vi "Create Sequence File.vi"(8 "error in (no error)":errorcluster, 11 "niRFSTS Sequence Flow in":refnum<class "niRFSTS Sequence Flow.lvclass">) -> (0 "error out":errorcluster, 3 "niRFSTS Sequence Flow out":refnum<class "niRFSTS Sequence Flow.lvclass">)   [LabVIEW 2018, in "niRFSTS Sequence Flow.lvclass"]
uses:
  niRFSTS Sequence Flow.lvclass
  niRFSTS Sequence Flow.lvclass/niRFSTS Sequence Flow.ctl
  Plugins/TestStand API Tools (TSAT).lvlibp/Sequence File Actions/TSAT Sequence File Actions.lvlib
  Plugins/TestStand API Tools (TSAT).lvlibp/TSAT Examples/TSAT Examples.lvlib
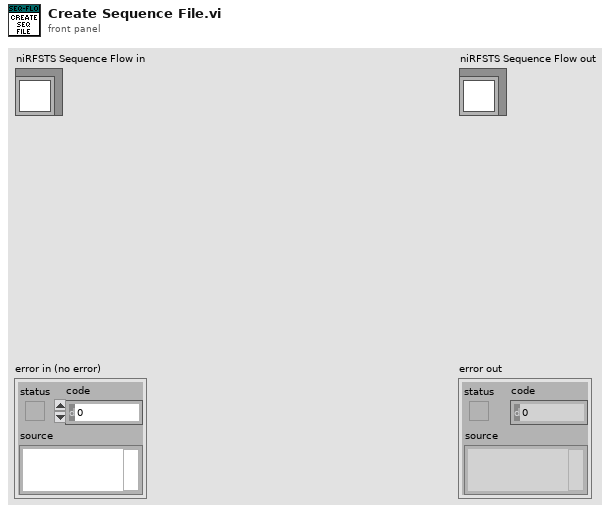
[diagram p1: front panel]
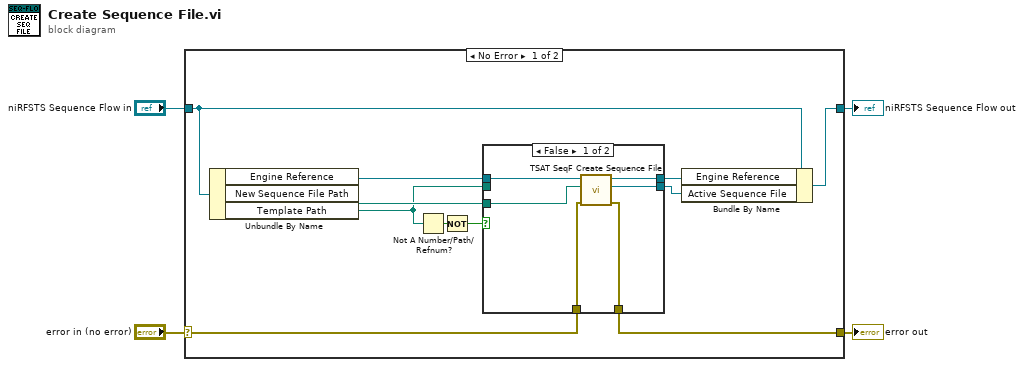
[diagram p0: block diagram]
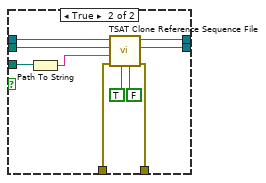
[diagram p2: hidden frame]
diagram:
  n1 = case shown="No Error" "error in (no error)" {
    selector: "error in (no error)" -> [w10 w33]
    tunnel: [w9 w33] -> w3
    tunnel: [w5 w32] -> w1
    tunnel: "niRFSTS Sequence Flow in" -> [w6 w32]
    frame No Error {
      n2 = Unbundle By Name(w6) -> ("Engine Reference"=w15:refnum<k7>, "New Sequence File Path"=w12:path, "Template Path"=w11:path)
      n3 = Not A Number/Path/Refnum?(number/path/refnum=w11) -> (NaN/Path/Refnum?=w14:bool)
      n4 = Not(x=w14) -> (.not. x?=w13:bool)
      n5 = case shown="False" w13 {
        tunnel: w15 -> [w21 w31]
        tunnel: w12 -> [w20 w24]
        tunnel: w10 -> [w19 w29]
        tunnel: [w18 w28] -> w9
        tunnel: [w17 w26] -> w7
        tunnel: [w16 w27] -> w8
        tunnel: w11 -> [_ w30]
        frame False {
          n6 = call "TSAT SeqF Create Sequence File.vi"("Error In"=w19, "Sequence File Location"=w20, "Engine In"=w21) -> ("Error Out"=w18:errorcluster, "Sequence File"=w17:refnum<k7>, "Engine Out"=w16:refnum<k7>)  [unwired: 6 in]
        }
        frame True {
          n7 = Path To String(path=w24) -> (string=w23:string)
          n8 = call "TSAT Clone Reference Sequence File.vi"("Save Reference File?(T)"=FALSE ("Save Sequence File?(T)"), "Specify Path"=TRUE, "Error In"=w29, "New File Name"=w23, "Sequence File Path"=w30, "Engine In"=w31) -> ("Error Out"=w28:errorcluster, "New Sequence File Out"=w26:refnum<k7>, "Engine out"=w27:refnum<k7>)  [unwired: 3 in]
        }
      }
      n9 = Bundle By Name(cluster=w6, "Engine Reference"=w8, "Active Sequence File"=w7) -> (w5:refnum<class "niRFSTS Sequence Flow.lvclass">)
    }
    frame Error {
    }
  }
  "error out" <- w3
  "niRFSTS Sequence Flow out" <- w1
